vi "plot_clear_weather.vi"(2 "Clearing Array":dbl[](array[numeric]), 5 "Buffer Size":dbl=1800.0, 9 "Input Arrays":dbl[][](array[numeric])=[[1.0, 4.0, 7.0], [2.0, 5.0, 8.0], [3.0, 6.0, 9.0]]) -> (10 "Output Arrays":dbl[][](array[numeric]))   [LabVIEW 2018]
doc: "Adds the datapoints for Timestamp, Rain Rate, and Accumulation to their corresponding plot arrays."
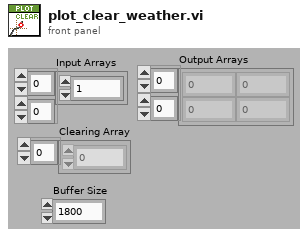
[diagram p1: front panel]
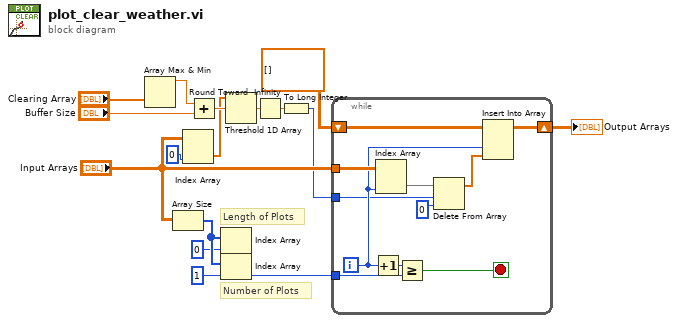
[diagram p0: block diagram]
diagram:
  # "Number of Plots"
  # "Length of Plots"
  n1 = Array Max & Min(array="Clearing Array") -> (max value=w10:dbl)  [unwired: 3 out]
  n2 = Array Size(array="Input Arrays") -> (size(s)=w16:i32[])
  n3 = Index Array(array="Input Arrays", index (col)=0 ("disabled index (col)")) -> (element=w2:dbl[])  [unwired: 1 in]
  n4 = Add(x=w10, y="Buffer Size") -> (x+y=w5:dbl)
  n5 = Index Array(array=w16, index=0) -> ()  [unwired: 1 out]
  n6 = Index Array(array=w16, index=1) -> (element=w15:i32)
  n7 = Threshold 1D Array(2:w5, 3:w2) -> (0:w7:dbl)  [unwired: 1 in]
  n8 = Round Toward -Infinity(1:w7) -> (0:w6:dbl)
  n9 = To Long Integer(number=w6) -> (32bit integer=w1:i32)
  n10 = while {
    tunnel: w15 -> [w24]
    tunnel: "Input Arrays" -> [w27]
    shift-right: [w26] -> w12
    shift-left: dbl[][] [] ("Plot Arrays") -> [w25]
    tunnel: w1 -> [w17]
    i -> [w21]
    stop <- w23 stop-if-true
    n11 = Increment(x=w21) -> (x+1=w22:i32)
    n12 = Index Array(array=w27, index (col)=w21) -> (element=w19:dbl[])  [unwired: 1 in]
    n13 = Greater Or Equal?(x=w22, y=w24) -> (x >= y?=w23:bool)
    n14 = Delete From Array(array=w19, length=w17, index=0) -> (array with subset deleted=w18:dbl[])  [unwired: 1 out]
    n15 = Insert Into Array(array=w25, index (col)=w21, new element=w18) -> (w26:dbl[][])  [unwired: 1 in]
  }
  "Output Arrays" <- w12
